vi "Configure Trigger.vi"(0 "VISA resource name":refnum<visa-resource-name>, 1 "Trigger Level (0dBm)":i32 min=-150 max=50, 5 "Trigger Delay (20.000000ms)":dbl=20.0 min=-1000.0 max=1000.0 format="%.6f", 7 "Trigger Mode (0:Free Run)":i32(ring) items=["Free Run", "Triggered"], 9 "Trigger Source (0:Video Trigger)":i32(ring) items=["Video Trigger", "Wide IF Video", "External Trigger", "SG Marker Trigger"], 11 "error in (no error)":errorcluster, 12 "Trigger Edge (0:Rise)":i32(ring) items=["Rise", "Fall"]) -> (4 "VISA resource name out":refnum<visa-resource-name>, 15 "error out":errorcluster)   [LabVIEW 2020, in "Anritsu Signal Analyzer Series.lvlib"]
doc: "Configures the trigger settings of the spectrum analyzer."
uses:
  Anritsu Signal Analyzer Series.lvlib
panel:
  # "dBm"
  # "ms"
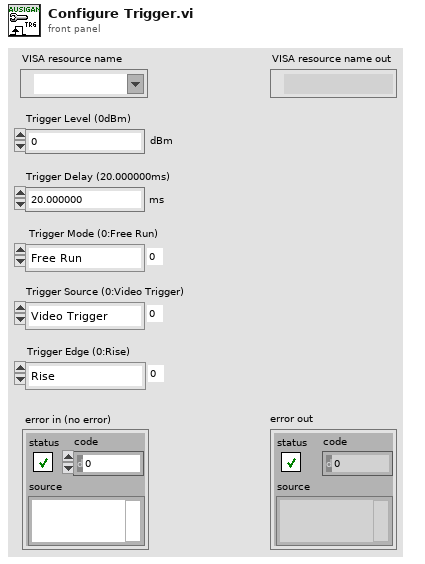
[diagram p1: front panel]
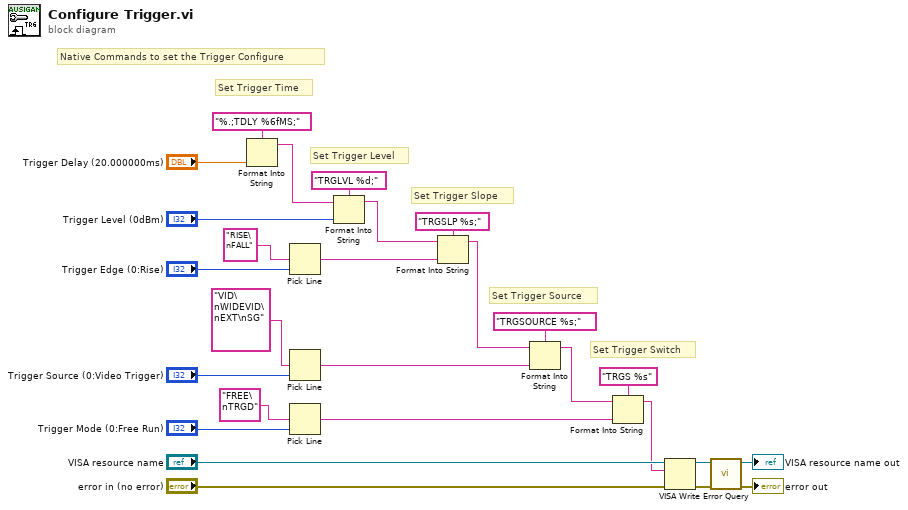
[diagram p0: block diagram]
diagram:
  # "Native Commands to set the Trigger Configure"
  # "Set Trigger Switch"
  # "Set Trigger Source"
  # "Set Trigger Slope"
  # "Set Trigger Level"
  # "Set Trigger Time"
  n1 = Format Into String(format string="%.;TDLY %6fMS;" ("Format String"), "Trigger Delay (20.000000ms)") -> (resulting string=w17:string)  [unwired: 2 in, 1 out]
  n2 = Pick Line(multi-line string="RISE\nFALL" ("複数行文字列"), line index="Trigger Edge (0:Rise)") -> (output string=w6:string)  [unwired: 1 in]
  n3 = Pick Line(multi-line string="VID\nWIDEVID\nEXT\nSG" ("複数行文字列"), line index="Trigger Source (0:Video Trigger)") -> (output string=w4:string)  [unwired: 1 in]
  n4 = Pick Line(multi-line string="FREE\nTRGD" ("複数行文字列"), line index="Trigger Mode (0:Free Run)") -> (output string=w2:string)  [unwired: 1 in]
  n5 = Format Into String(format string="TRGLVL %d;" ("Format String"), initial string=w17, "Trigger Level (0dBm)") -> (resulting string=w16:string)  [unwired: 1 in, 1 out]
  n6 = Format Into String(format string="TRGSLP %s;" ("_CommandSet"), initial string=w16, w6) -> (resulting string=w14:string)  [unwired: 1 in, 1 out]
  n7 = Format Into String(format string="TRGSOURCE %s;" ("_CommandSet"), initial string=w14, w4) -> (resulting string=w12:string)  [unwired: 1 in, 1 out]
  n8 = Format Into String(format string="TRGS %s" ("_CommandSet"), initial string=w12, w2) -> (resulting string=w8:string)  [unwired: 1 in, 1 out]
  n9 = VISA Write(VISA resource name="VISA resource name", write buffer=w8, error in (no error)="error in (no error)") -> (VISA resource name out=w9:refnum<visa-resource-name>, error out=w10:errorcluster)  [unwired: 1 out]
  n10 = call "Error Query.vi"("error in (no error)"=w10, "VISA resource name"=w9) -> ("error out"=→"error out":errorcluster, "VISA resource name out"=→"VISA resource name out":refnum<visa-resource-name>)  [unwired: 6 in, 2 out]
